vi "CO MFR sw 1.vi"(9 "Bottle conc":dbl, 10 "C_CO":dbl, 11 "Flow rate":dbl) -> (3 "CO MFR":dbl)   [LabVIEW 2014]
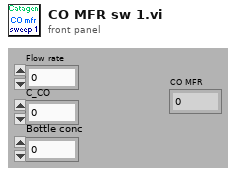
[diagram p1: front panel]
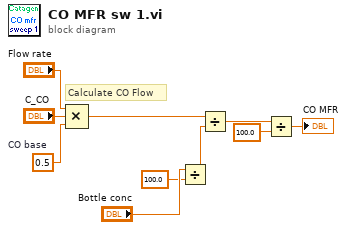
[diagram p0: block diagram]
diagram:
  w6 = 0.5  # CO base
  # "Calculate CO Flow"
  n1 = Compound Arithmetic op=MULTIPLY("Flow rate", "C_CO", w6) -> (w5:dbl)
  n2 = Divide(x="Bottle conc", y=100.0) -> (x/y=w1:dbl)
  n3 = Divide(x=w5, y=w1) -> (x/y=w4:dbl)
  n4 = Divide(x=w4, y=100.0) -> (x/y=→"CO MFR":dbl)
